vi "Check.vi"() -> ()   [LabVIEW 2019]
uses:
  YQ.xctl
  Y_state.ctl
  95228b63-dbad-4f81-a48d-2b4403cca3b5.vi
  Heating.lvlib
panel:
  in  "Y_State":T1=enum."hand"
  in  "Y":dbl
  out "Numeric":dbl
  in  "connect":bool
  in  "Y_control":dbl(xcontrol)
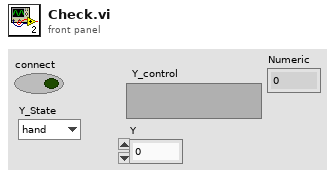
[diagram p1: front panel]
types:
  T1 = typedef "Heating.lvlib/Y_state.ctl" = enum8{"initialize", "alarm", "min", "stop", "hand", "auto", "max"}
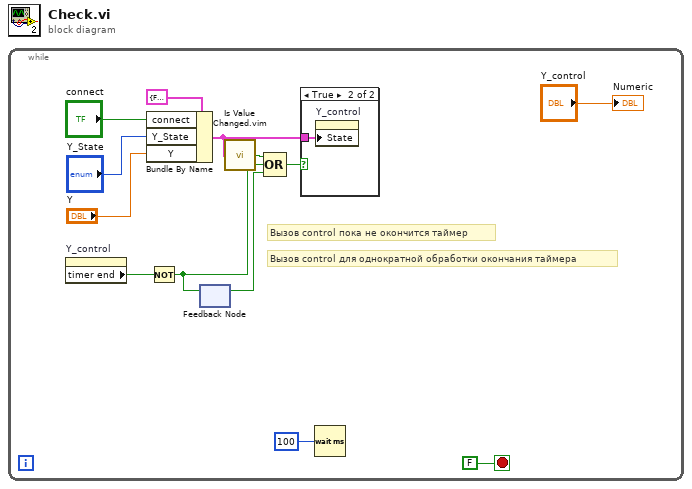
[diagram p0: block diagram]
diagram:
  n1 = while {
    stop <- FALSE stop-if-true
    # "Вызов control пока не окончится таймер"
    # "Вызов control для однократной обработки окончания таймера"
    n2 = property on="Y_control" class="YQ (strict)"() -> ("timer end"=w10:bool)  [unwired: 2 in, 2 out]
    n3 = Bundle By Name(cluster=cluster{"connect":bool, "Y_State":T1, "Y":dbl} {"connect"=FALSE, "Y_State"=enum."initialize", "Y"=0.0} ("source"), "connect"="connect", "Y_State"="Y_State", "Y"="Y") -> (w3:cluster{"connect":bool, "Y_State":T1, "Y":dbl})
    n4 = Not(x=w10) -> (.not. x?=w8:bool)
    n5 = feedback-in #1(w8) -> ()
    n6 = feedback #1() -> (w9:bool)  [unwired: 1 in]
    n7 = call "Is Value Changed.vim"("value"=w3) -> ("changed or first call?"=w2:bool)
    n8 = Compound Arithmetic op=OR(w2, w8, w9) -> (w11:bool)
    n9 = case shown="True" w11 {
      tunnel: w3 -> [_ w14]
      frame False {
      }
      frame True {
        n10 = property on="Y_control" class="YQ (strict)"("State"=w14) -> ()  [unwired: 2 in, 2 out]
      }
    }
    n11 = Wait (ms)(milliseconds to wait=u32 100) -> ()  [unwired: 1 out]
    "Numeric" <- "Y_control"
  }
